vi "File.Search for Files in a Folder.vi"(9 "Pattern":string, 11 "Dir":path) -> (1 "Match":bool, 3 "Matched Files":path[](array[path]))   [LabVIEW 2018]
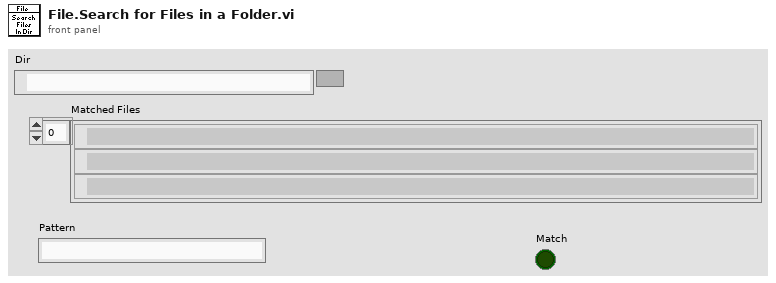
[diagram p1: front panel]
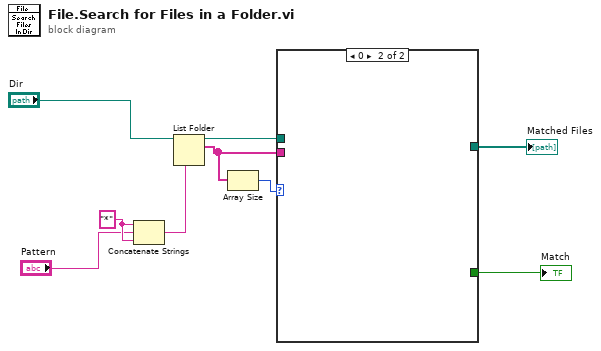
[diagram p0: block diagram]
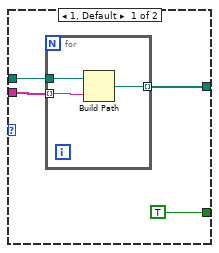
[diagram p2: hidden frame]
diagram:
  w9 = "*"
  n1 = Concatenate Strings(w9, "Pattern", w9) -> (w6:string)
  n2 = List Folder(path="Dir", pattern=w6) -> (path out=w4:path, filenames=w3:string[])  [unwired: 2 in, 2 out]
  n3 = Array Size(array=w3) -> (size(s)=w5:i32)
  n4 = case shown="0" w5 {
    tunnel: w4 -> [w13 _]
    tunnel: w3 -> [w12 _]
    tunnel: [w11 _] -> w2
    tunnel: [TRUE _] -> w1
    frame 1, Default {
      n5 = for {
        tunnel: w13 -> [w15]
        tunnel: w12 -> [w16] mode=indexing
        tunnel: [w14] -> w11 mode=indexing
        n6 = Build Path(base path=w15, name or relative path=w16) -> (appended path=w14:path)
      }
    }
    frame 0 {
    }
  }
  "Matched Files" <- w2
  "Match" <- w1
